vi "CALC_Angle_of_the_rotation_of_the_cage_itself_(arr).vi"(1 "Y1-Y2":dbl[](array[numeric]), 2 "X1-X2":dbl[](array[numeric]), 3 "sin(a)":dbl[](array[numeric])) -> (0 "Cage rot. angle, rad":dbl[](array[numeric]))   [LabVIEW 2018, in "Tracker.lvlib"]
uses:
  Tracker.lvlib
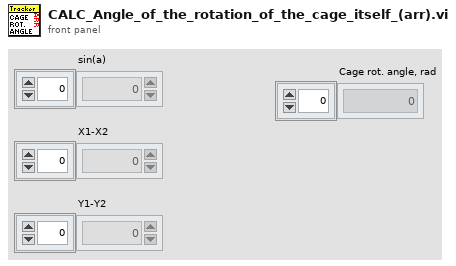
[diagram p1: front panel]
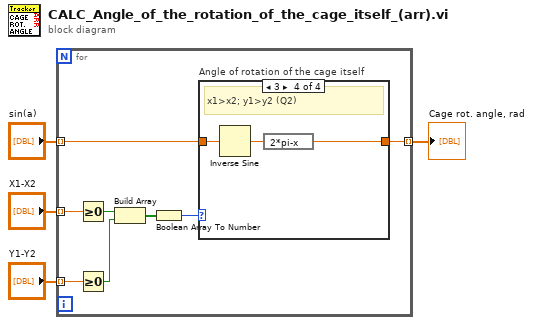
[diagram p0: block diagram]
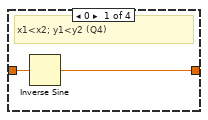
[diagram p2: hidden frame]
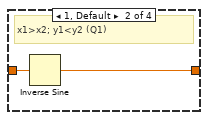
[diagram p3: hidden frame]
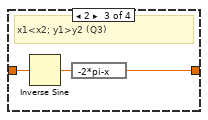
[diagram p4: hidden frame]
diagram:
  n1 = for {
    tunnel: "X1-X2" -> [w8] mode=indexing
    tunnel: "Y1-Y2" -> [w7] mode=indexing
    tunnel: "sin(a)" -> [w6] mode=indexing
    tunnel: [w5] -> w1 mode=indexing
    n2 = Greater Or Equal To 0?(x=w8) -> (x >= 0?=w9:bool)
    n3 = Greater Or Equal To 0?(x=w7) -> (x >= 0?=w10:bool)
    n4 = Build Array(w9, w10) -> (w11:bool[])
    n5 = Boolean Array To Number(Boolean array=w11) -> (number=w12:u32)
    n6 = case "Angle of rotation of the cage itself" shown="3" w12 {
      tunnel: w6 -> [w14 w16 w18 w21]
      tunnel: [w13 w15 w17 w20] -> w5
      frame 0 {
        # "x1<x2; y1<y2 (Q4)"
        n7 = Inverse Sine(1:w14) -> (0:w13:dbl)
      }
      frame 1, Default {
        # "x1>x2; y1<y2 (Q1)"
        n8 = Inverse Sine(1:w16) -> (0:w15:dbl)
      }
      frame 2 {
        # "x1<x2; y1>y2 (Q3)"
        n9 = Inverse Sine(1:w18) -> (0:w19:dbl)
        n10 = expression code="-2*pi-x" ("radians to degrees")(w19) -> (w17:dbl)
      }
      frame 3 {
        # "x1>x2; y1>y2 (Q2)"
        n11 = Inverse Sine(1:w21) -> (0:w22:dbl)
        n12 = expression code="2*pi-x" ("radians to degrees")(w22) -> (w20:dbl)
      }
    }
  }
  "Cage rot. angle, rad" <- w1
